vi "Build Ymodem data frame.vi"(9 "Data Index(1)":u8=1, 11 "Data Buffer":string) -> (3 "Frame Data":u8[](array[numeric]) format="%02x")   [LabVIEW 2013]
doc: "Build the data body part(1204 bytes or 128 bytes) of the YModem protocol."
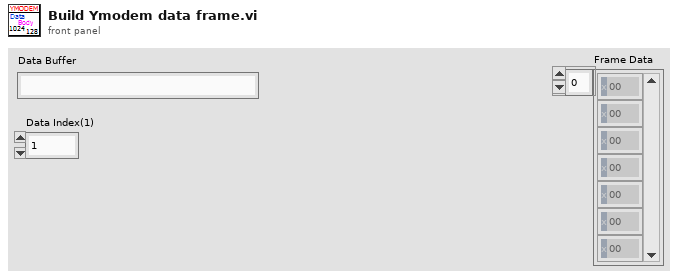
[diagram p1: front panel]
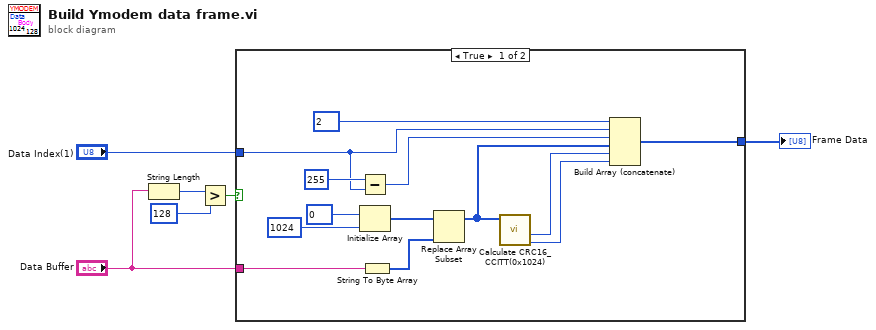
[diagram p0: block diagram]
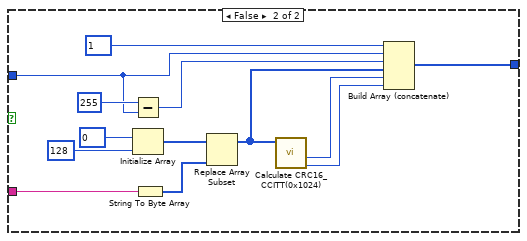
[diagram p2: hidden frame]
diagram:
  n1 = String Length(string="Data Buffer") -> (length=w3:i32)
  n2 = Greater?(x=w3, y=128) -> (0:w1:bool)
  n3 = case shown="True" w1 {
    tunnel: "Data Index(1)" -> [w18 w31]
    tunnel: [w12 w25] -> w5
    tunnel: "Data Buffer" -> [w11 w24]
    frame True {
      n4 = Subtract(x=u8 255 ("Numeric"), y=w18) -> (x-y=w17:u8)
      n5 = Initialize Array(u8 0 ("Numeric"), 1024 ("dimension size")) -> (w14:u8[])
      n6 = String To Byte Array(string=w11) -> (unsigned byte array=w13:u8[])
      n7 = Replace Array Subset(array=w14, new element=w13) -> (w9:u8[])  [unwired: 1 in]
      n8 = call "Calculate CRC16_CCITT(0x1024).vi"("Data in"=w9) -> ("Lo CRC16"=w7:u8, "Hi CRC16"=w8:u8)  [unwired: 7 in, 2 out]
      n9 = Build Array (concatenate)(u8 2 ("Numeric"), w18, w17, w9, w8, w7) -> (w12:u8[])
    }
    frame False {
      n10 = Subtract(x=u8 255 ("Numeric"), y=w31) -> (x-y=w30:u8)
      n11 = Initialize Array(u8 0 ("Numeric"), 128 ("dimension size")) -> (w27:u8[])
      n12 = String To Byte Array(string=w24) -> (unsigned byte array=w26:u8[])
      n13 = Replace Array Subset(array=w27, new element=w26) -> (w22:u8[])  [unwired: 1 in]
      n14 = call "Calculate CRC16_CCITT(0x1024).vi"("Data in"=w22) -> ("Lo CRC16"=w20:u8, "Hi CRC16"=w21:u8)  [unwired: 7 in, 2 out]
      n15 = Build Array (concatenate)(u8 1 ("Numeric"), w31, w30, w22, w21, w20) -> (w25:u8[])
    }
  }
  "Frame Data" <- w5
